vi "Open.vi"(4 "Max Value":dbl[](array[numeric]), 6 "Min Value":dbl[](array[numeric]), 8 "error in (no error)":errorcluster, 10 "Channel Names":tag[](array[tag])) -> (0 "error out":errorcluster, 3 "AI (Continuous) Ref Out":T1)   [LabVIEW 2021, in "AI Continuous.lvlib"]
uses:
  <vilib>/myRIO/Instrument Drivers/Onboard IO/AI Continuous/AI Continuous.lvlib
  <vilib>/myRIO/Instrument Drivers/Onboard IO/AI Continuous/typedefs/AI Continuous Reference.ctl
  <vilib>/myRIO/Common/Instrument Driver Framework/Utilities/typedefs/myRIO Generic Hardware Reference.ctl
  <vilib>/myRIO/Common/Instrument Driver Framework/Utilities/typedefs/Hardware Version Enum.ctl
  <vilib>/myRIO/Common/Instrument Driver Framework/Utilities/typedefs/myRIO v1.0 Reference.ctl
  <vilib>/myRIO/Common/Instrument Driver Framework/Utilities/typedefs/Generic FPGA Reference.ctl
  <vilib>/myRIO/Common/Instrument Driver Framework/ELVIS III v1.0/AI Continuous/typedefs/AI Continuous Channels List.ctl
  <vilib>/myRIO/Common/Instrument Driver Framework/ELVIS III v1.0/AI Continuous/typedefs/ELVIS III v1.0 AI Continuous Channels Enum.ctl
  <vilib>/myRIO/Common/Instrument Driver Framework/Utilities/typedefs/Analog Scaling Constants.ctl
  <vilib>/userdefined/High Color/nirio_resource_hc.ctl
panel:
  # "AI (Continuous) Open"
  # "Opens a reference to the myRIO hardware and configures the AI Continuous Reference with channels to be read"
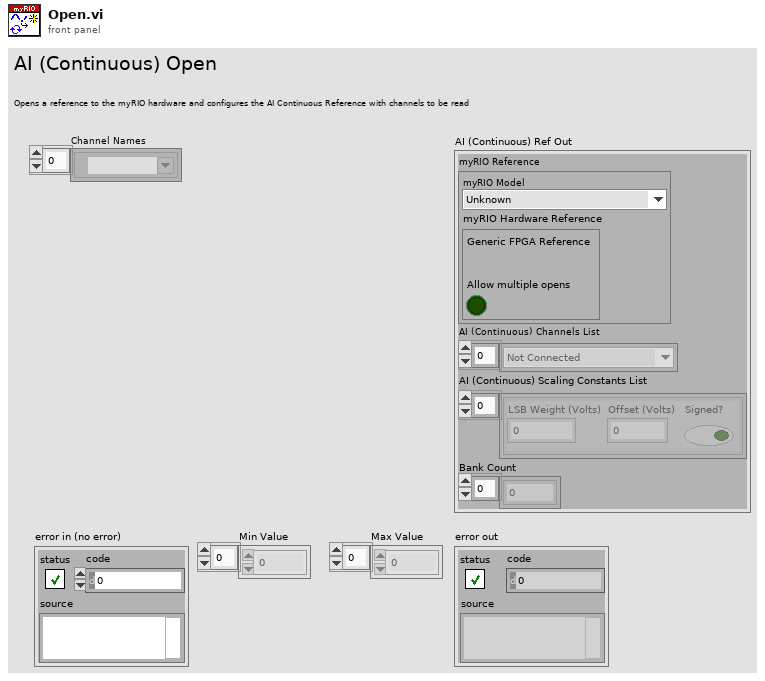
[diagram p1: front panel]
types:
  T1 = typedef "AI Continuous.lvlib/AI Continuous Reference.ctl" = cluster{"myRIO Reference":T2, "AI (Continuous) Channels List":T6, "AI (Continuous) Scaling Constants List":T8[], "Bank Count":u8[]}
  T2 = typedef "myRIO Generic Hardware Reference.ctl" = cluster{"myRIO Model":T3, "myRIO Hardware Reference":T4}
  T3 = typedef "Hardware Version Enum.ctl" = enum16{"Unknown", "myRIO-1900", "myRIO-1950", "roboRIO", "NI ELVIS RIO CM", "ELVIS III"}
  T4 = typedef "myRIO v1.0 Reference.ctl" = cluster{"Generic FPGA Reference":T5, "Allow multiple opens":bool}
  T5 = typedef "Generic FPGA Reference.ctl" = refnum<k20>
  T6 = typedef "AI Continuous Channels List.ctl" = T7[]
  T7 = typedef "ELVIS III v1.0 AI Continuous Channels Enum.ctl" = enum16{"Not Connected", "A/AI0 (Continuous)", "A/AI1 (Continuous)", "A/AI2 (Continuous)", "A/AI3 (Continuous)", "A/AI4 (Continuous)", "A/AI5 (Continuous)", "A/AI6 (Continuous)", "A/AI7 (Continuous)", "A/AI0 (DIFF Continuous)", "A/AI1 (DIFF Continuous)", "A/AI2 (DIFF Continuous)", "A/AI3 (DIFF Continuous)", "B/AI0 (Continuous)", "B/AI1 (Continuous)", "B/AI2 (Continuous)", "B/AI3 (Continuous)", "B/AI4 (Continuous)", "B/AI5 (Continuous)", "B/AI6 (Continuous)", "B/AI7 (Continuous)", "B/AI0 (DIFF Continuous)", "B/AI1 (DIFF Continuous)", "B/AI2 (DIFF Continuous)", "B/AI3 (DIFF Continuous)"}
  T8 = typedef "Analog Scaling Constants.ctl" = cluster{"LSB Weight (Volts)":dbl, "Offset (Volts)":dbl, "Signed?":bool}
  T9 = typedef "nirio_resource_hc.ctl" = tag
  T10 = typedef "Analog Scaling Constants List.ctl" = T8[]
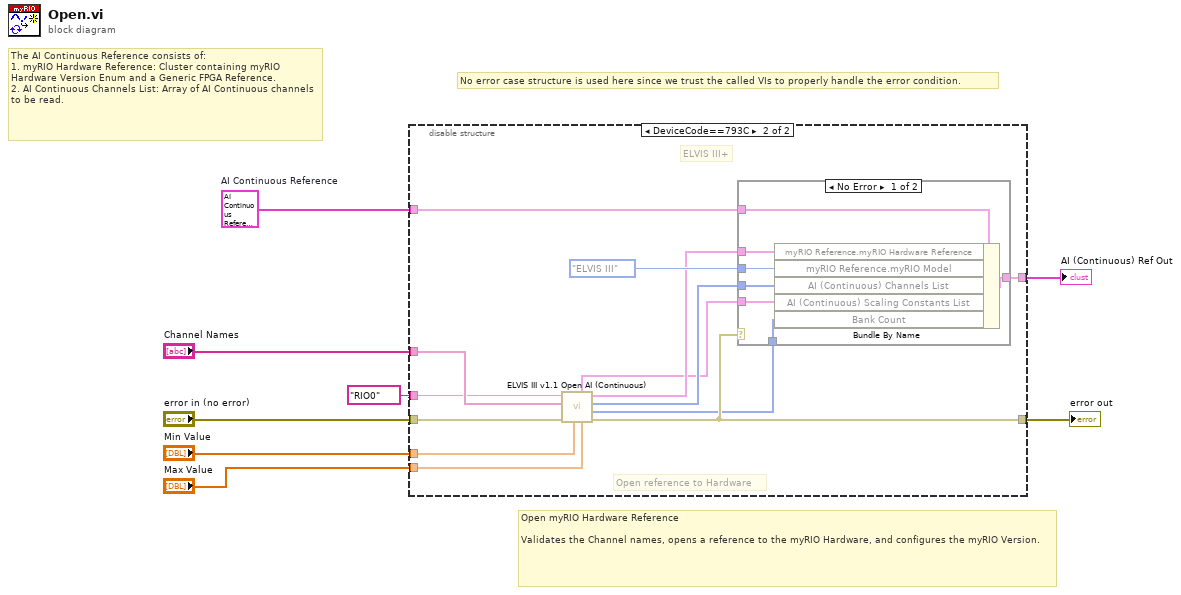
[diagram p0: block diagram]
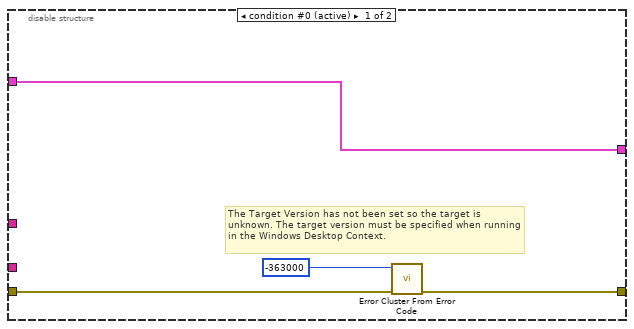
[diagram p2: hidden frame]
diagram:
  w5 = T1 {"myRIO Reference"={"myRIO Model"=enum."Unknown", "myRIO Hardware Reference"={"Generic FPGA Reference"=refnum, "Allow multiple opens"=FALSE}}, "AI (Continuous) Channels List"=[], "AI (Continuous) Scaling Constants List"=[], "Bank Count"=[]}  # AI Continuous Reference
  # "No error case structure is used here since we trust the called VIs to properly handle the error condition."
  # "The AI Continuous Reference consists of:\n1. myRIO Hardware Reference: Cluster containing myRIO Hardware Version Enum and a Generic FPGA Reference.\n2. AI Continuous Channels List: Array of AI Continuous channels to be read."
  # "Open myRIO Hardware Reference\n\nValidates the Channel names, opens a reference to the myRIO Hardware, and configures the myRIO Version."
  n1 = disable-structure shown="DeviceCode==793C" {
    disable-tunnel: [w12 w14] -> w6
    disable-tunnel: "Channel Names" -> [_ w20]
    disable-tunnel: [w9 w15] -> w1
    disable-tunnel: "error in (no error)" -> [w11 w18]
    disable-tunnel: w5 -> [w9 w21]
    disable-tunnel: T9 "RIO0" ("Resource name") -> [_ w19]
    disable-tunnel: "Min Value" -> [_ w17]
    disable-tunnel: "Max Value" -> [_ w16]
    frame condition #0 (active) {
      # "The Target Version has not been set so the target is unknown. The target version must be specified when running in the Windows Desktop Context."
      n2 = call <vilib>:"Error Cluster From Error Code.vi"("error in (no error)"=w11, "error code (0)"=-363000) -> ("error out"=w12:errorcluster)  [unwired: 7 in]
    }
    frame condition #1 {
      # "ELVIS III+"
      # "Open reference to Hardware"
      n3 = call <vilib>:"ELVIS III v1.1 Open AI (Continuous).vi"("Max Value"=w16, "Min Value"=w17, "error in (no error)"=w18, "Channel Names"=w20, "Resource name"=w19) -> ("error out"=w14:errorcluster, "Bank Count"=w13:u8[], "AI (Continuous) Channels List"=w23:T6, "AI (Continuous) Ref Out"=w24:T4, "AI (Continous) Read Scale Constants List"=w22:T10)  [unwired: 2 in]
      n4 = case shown="No Error" w14 {
        tunnel: [w32 w33] -> w15
        tunnel: Hardware_Version_Enum."ELVIS III" ("Hardware Version Enum") -> [w31 _]
        tunnel: w24 -> [w29 _]
        tunnel: w21 -> [w30 w33]
        tunnel: w23 -> [w27 _]
        tunnel: w22 -> [w28 _]
        tunnel: w13 -> [w26 _]
        frame No Error {
          n5 = Bundle By Name(cluster=w30, "myRIO Reference.myRIO Hardware Reference"=w29, "myRIO Reference.myRIO Model"=w31, "AI (Continuous) Channels List"=w27, "AI (Continuous) Scaling Constants List"=w28, "Bank Count"=w26) -> (w32:T1)
        }
        frame Error {
        }
      }
    }
  }
  "error out" <- w6
  "AI (Continuous) Ref Out" <- w1
